vi "New.vi"(8 "error in (no error)":errorcluster, 9 "Type":string, 10 "Parent":refnum<class "Config Element.lvclass">, 11 "Name":string) -> (0 "error out":errorcluster, 3 "Task out":refnum<class "Task.lvclass">)   [LabVIEW 2020, in "VolatusConfig.lvlib" / "Task.lvclass"]
uses:
  Task.lvclass
  lv-cdm/CDM-Config/Config Element/Config Element.lvclass
  Task.lvclass/Task.ctl
  lv-cdm/CDM-Config/Value Type.ctl
  lv-cdm/CDM-Config/CDM-Config.lvlib
  VolatusConfig.lvlib
  Meta Type.ctl
  Meta Name.ctl
  VolatusConfigElement/VolatusConfigElement.lvclass
  C:/dev/lv20CE/relink/lv-volatus/VolatusConfig/VolatusConfigElement/VolatusConfigElement.lvclass
  C:/dev/lv20CE/relink/lv-volatus/VolatusConfig/Task/Task.lvclass
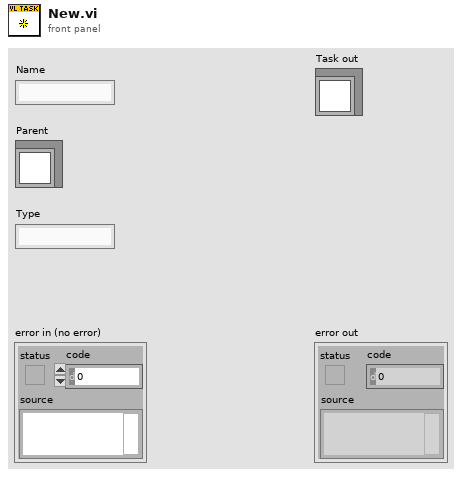
[diagram p1: front panel]
types:
  T1 = typedef "VolatusConfig.lvlib/Meta Name.ctl" = enum16{"VL_Type", "VL_Node_IP", "VL_Node_Type", "VL_Task_Type", "VL_Group_Type", "VL_Channel_Type", "VL_Channel_DataType", "VL_Config_Version", "VL_Overlay_Type"}
  T2 = typedef "VolatusConfig.lvlib/Meta Type.ctl" = enum16{"UNKNOWN", "VL_System", "VL_Cluster", "VL_Node", "VL_Task", "VL_Group", "VL_Channel", "VL_Task_List", "VL_Scaling", "VL_Sensor", "VL_Sensor_List", "VL_Scale"}
  T3 = typedef "CDM-Config.lvlib/Value Type.ctl" = enum16{"String", "Number", "Bool", "Object", "Array"}
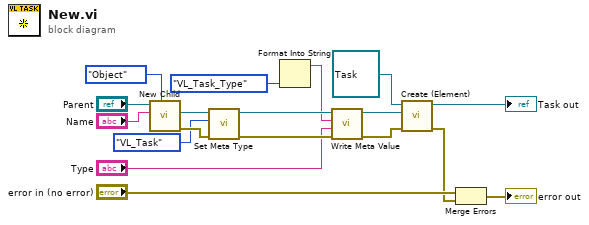
[diagram p0: block diagram]
diagram:
  n1 = call "New Child.vi"("Value Type (String)"=Value_Type."Object", "Child Name"="Name", "Config Element in"="Parent") -> ("error out"=w12:errorcluster, "New Child"=w13:refnum<class "Config Element.lvclass">)  [unwired: 6 in, 1 out]
  n2 = call "Set Meta Type.vi"("error in (no error)"=w12, "Meta Type"=Meta_Type."VL_Task", "Element In"=w13) -> ("error out"=w9:errorcluster, "Element"=w10:refnum<class "Config Element.lvclass">)  [unwired: 7 in]
  n3 = Format Into String(Meta_Name."VL_Task_Type" ("Meta Name")) -> (resulting string=w7:string)  [unwired: 3 in, 1 out]
  n4 = call "Write Meta Value.vi"("error in (no error)"=w9, "Meta Value"="Type", "Meta Name"=w7, "Config Element in"=w10) -> ("error out"=w3:errorcluster, "Config Element out"=w4:refnum<class "Config Element.lvclass">)  [unwired: 6 in]
  n5 = call "Create (Element).vi"("error in (no error)"=w3, "Element"=w4, "VolatusConfigElement in"=refnum<class "Task.lvclass"> refnum ("Task in")) -> ("error out"=w1:errorcluster, "VolatusConfigElement out"=→"Task out":refnum<class "Task.lvclass">)  [unwired: 7 in]
  n6 = Merge Errors("error in (no error)", w1) -> (→"error out":errorcluster)
